vi "ControlFileToVariant.vi"(8 "error in":errorcluster, 11 "State":T1={"paths"={"index cluster path"=path "C:/Users/bcelis.AMER/Documents/TBDCore/source/Utilities/Cluster to Tag Bus Scripts/Controls/IndexCluster.ctl", "cluster path"=path "C:/Users/bcelis.AMER/Documents/TBDCore/source/Utilities/Cluster to Tag Bus Scripts/Controls/SampleControl.ctl", "cluster to tag bus VI path"=path "C:/Users/bcelis.AMER/Documents/TBDCore/source/Utilities/Cluster to Tag Bus Scripts/ClustertoTagbus.vi", " tag bus to cluster VI path"=path ""}, "write VI ref"=refnum, "read VI ref"=refnum, "base cluster"=variant, "vi refs"={"data ctl"=refnum, "index ctl"=refnum, "interface vi"=refnum, "vi type"=enum."tb to data"}}) -> (0 "error out":errorcluster, 3 "State out":T1={"paths"={"index cluster path"=path "C:/Users/bcelis.AMER/Documents/TBDCore/source/Utilities/Cluster to Tag Bus Scripts/Controls/IndexCluster.ctl", "cluster path"=path "C:/Users/bcelis.AMER/Documents/TBDCore/source/Utilities/Cluster to Tag Bus Scripts/Controls/SampleControl.ctl", "cluster to tag bus VI path"=path "C:/Users/bcelis.AMER/Documents/TBDCore/source/Utilities/Cluster to Tag Bus Scripts/ClustertoTagbus.vi", " tag bus to cluster VI path"=path ""}, "write VI ref"=refnum, "read VI ref"=refnum, "base cluster"=variant, "vi refs"={"data ctl"=refnum, "index ctl"=refnum, "interface vi"=refnum, "vi type"=enum."tb to data"}})   [LabVIEW 2013]
uses:
  Controls/StateCluster.ctl
  Controls/PathsCluster.ctl
  Controls/initialized references.ctl
  Controls/interface VI type.ctl
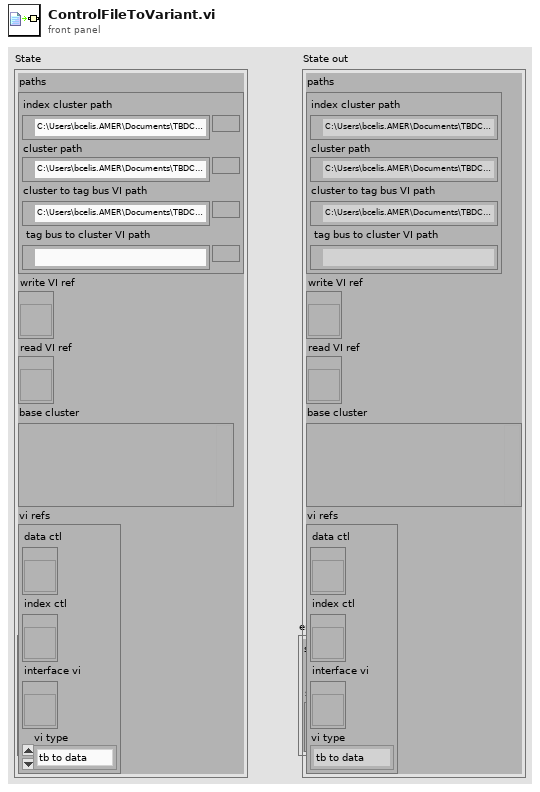
[diagram p1: front panel]
types:
  T1 = typedef "StateCluster.ctl" = cluster{"paths":T2, "write VI ref":refnum<vi>, "read VI ref":refnum<vi>, "base cluster":variant, "vi refs":T3}
  T2 = typedef "PathsCluster.ctl" = cluster{"index cluster path":path, "cluster path":path, "cluster to tag bus VI path":path, " tag bus to cluster VI path":path}
  T3 = typedef "initialized references.ctl" = cluster{"data ctl":refnum<vi>, "index ctl":refnum<vi>, "interface vi":refnum<vi>, "vi type":T4}
  T4 = typedef "interface VI type.ctl" = enum16{"tb to data", "data to tb"}
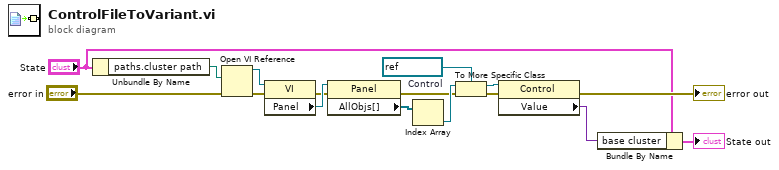
[diagram p0: block diagram]
diagram:
  w14 = refnum<vi> refnum  # Control
  n1 = Unbundle By Name("State") -> ("paths.cluster path"=w6:path)
  n2 = Open VI Reference(vi path=w6, error in (no error)="error in") -> (vi reference=w9:refnum<vi>, error out=w1:errorcluster)  [unwired: 4 in]
  n3 = property class="VI"(reference=w9, error in=w1) -> (error out=w7:errorcluster, "Panel"=w8:refnum<vi>)  [unwired: 1 out]
  n4 = property class="Panel"(reference=w8, error in=w7) -> (error out=w2:errorcluster, "AllObjs[]"=w10:refnum<vi>[])  [unwired: 1 out]
  n5 = Index Array(array=w10) -> (element=w12:refnum<vi>)  [unwired: 1 in]
  n6 = To More Specific Class(target class=w14, reference=w12, error in=w2) -> (specific class reference=w13:refnum<vi>, error out=w11:errorcluster)
  n7 = property class="Control"(reference=w13, error in=w11) -> (error out=→"error out":errorcluster, "Value"=w4:variant)  [unwired: 1 out]
  n8 = Bundle By Name(cluster="State", "base cluster"=w4) -> (→"State out":T1)
